vi "Analog Output Write Manual.vi"(8 "error in":errorcluster, 10 "Analog Output Write":dbl[](array[numeric]) format="%0.2f", 11 "NI Analog Output in":refnum<class "NI Analog Output.lvclass">) -> (0 "error out":errorcluster, 3 "NI Analog Output out":refnum<class "NI Analog Output.lvclass">)   [LabVIEW 2023, in "HardwareAbstractionLayer_LVOOP.lvlib" / "NI Analog Output.lvclass"]
uses:
  NI Analog Output.lvclass
  NI Analog Output.lvclass/NI Analog Output.ctl
  <vilib>/DAQmx/write.llb/DAQmx Write (Analog 1D DBL NChan 1Samp).vi
  <vilib>/DAQmx/miscellaneous.llb/DAQmx Fill In Error Info.vi
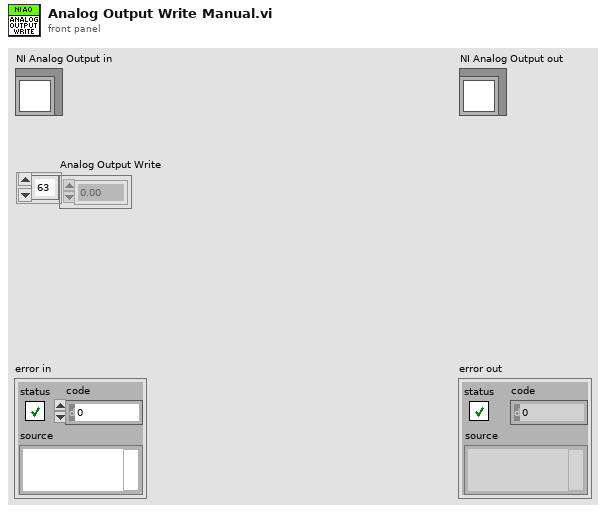
[diagram p1: front panel]
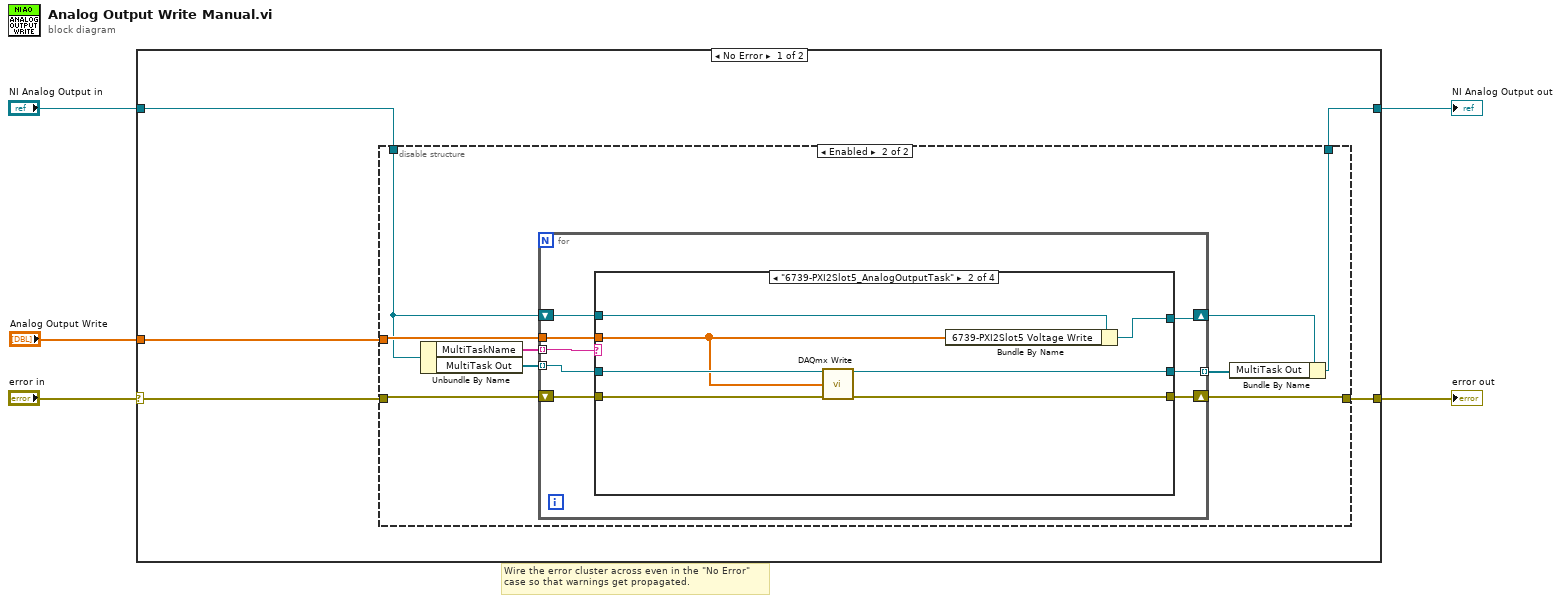
[diagram p0: block diagram]
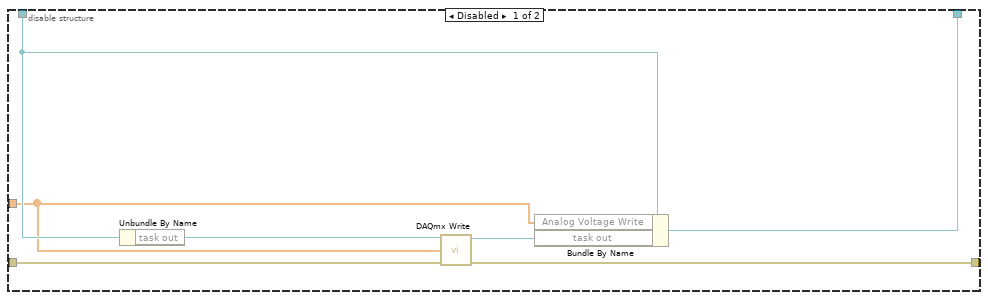
[diagram p2: hidden frame]
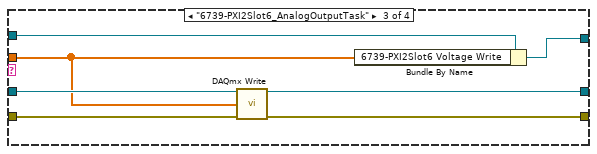
[diagram p4: hidden frame]
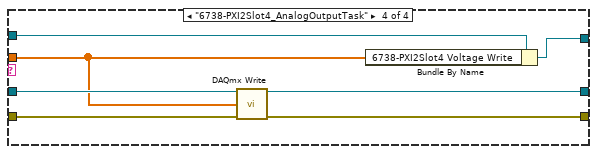
[diagram p5: hidden frame]
diagram:
  # "Wire the error cluster across even in the \"No Error\"\ncase so that warnings get propagated."
  n1 = case shown="No Error" "error in" {
    selector: "error in" -> [w10 w59]
    tunnel: [w9 w59] -> w4
    tunnel: [w7 w58] -> w2
    tunnel: "NI Analog Output in" -> [w8 w58]
    tunnel: "Analog Output Write" -> [w6 _]
    frame No Error {
      n2 = disable-structure shown="Enabled" {
        disable-tunnel: w10 -> [w17 w26]
        disable-tunnel: [w16 w25] -> w9
        disable-tunnel: w8 -> [w15 w21]
        disable-tunnel: [w14 w19] -> w7
        disable-tunnel: w6 -> [w11 w24]
        frame Disabled {
          n3 = Unbundle By Name(w15) -> ("task out"=w12:refnum<k21>)
          n4 = call-poly <vilib>:"DAQmx Write.vi"("task/channels in"=w12, "data"=w11, "error in"=w17) -> ("task out"=w13:refnum<k21>, "error out"=w16:errorcluster)  [unwired: 10 in, 1 out]
          n5 = Bundle By Name(cluster=w15, "Analog Voltage Write"=w11, "task out"=w13) -> (w14:refnum<class "NI Analog Output.lvclass">)
        }
        frame Enabled {
          n6 = Unbundle By Name(w21) -> ("MultiTaskName"=w23:string[], "MultiTask Out"=w22:refnum<k21>[])
          n7 = for {
            tunnel: w24 -> [w32]
            shift-right: [w33] -> w25
            shift-left: w26 -> [w34]
            tunnel: w23 -> [w31] mode=indexing
            tunnel: w22 -> [w30] mode=indexing
            shift-right: [w28] -> w20
            shift-left: w21 -> [w29]
            tunnel: [w27] -> w18 mode=indexing
            n8 = case shown="\"6739-PXI2Slot5_AnalogOutputTask\"" w31 {
              tunnel: w34 -> [w36 w43 w50 w57]
              tunnel: [w36 w42 w49 w56] -> w33
              tunnel: w32 -> [_ w37 w44 w51]
              tunnel: w30 -> [_ w41 w48 w55]
              tunnel: w29 -> [w35 w40 w47 w54]
              tunnel: [w35 w39 w46 w53] -> w28
              tunnel: [_ w38 w45 w52] -> w27
              frame "", Default {
              }
              frame "6739-PXI2Slot5_AnalogOutputTask" {
                n9 = call-poly <vilib>:"DAQmx Write.vi"("task/channels in"=w41, "data"=w37, "error in"=w43) -> ("task out"=w38:refnum<k21>, "error out"=w42:errorcluster)  [unwired: 10 in, 1 out]
                n10 = Bundle By Name(cluster=w40, "6739-PXI2Slot5 Voltage Write"=w37) -> (w39:refnum<class "NI Analog Output.lvclass">)
              }
              frame "6739-PXI2Slot6_AnalogOutputTask" {
                n11 = call-poly <vilib>:"DAQmx Write.vi"("task/channels in"=w48, "data"=w44, "error in"=w50) -> ("task out"=w45:refnum<k21>, "error out"=w49:errorcluster)  [unwired: 10 in, 1 out]
                n12 = Bundle By Name(cluster=w47, "6739-PXI2Slot6 Voltage Write"=w44) -> (w46:refnum<class "NI Analog Output.lvclass">)
              }
              frame "6738-PXI2Slot4_AnalogOutputTask" {
                n13 = call-poly <vilib>:"DAQmx Write.vi"("task/channels in"=w55, "data"=w51, "error in"=w57) -> ("task out"=w52:refnum<k21>, "error out"=w56:errorcluster)  [unwired: 10 in, 1 out]
                n14 = Bundle By Name(cluster=w54, "6738-PXI2Slot4 Voltage Write"=w51) -> (w53:refnum<class "NI Analog Output.lvclass">)
              }
            }
          }
          n15 = Bundle By Name(cluster=w20, "MultiTask Out"=w18) -> (w19:refnum<class "NI Analog Output.lvclass">)
        }
      }
    }
    frame Error {
    }
  }
  "error out" <- w4
  "NI Analog Output out" <- w2
